vi "Dec 2.vi"() -> ()   [LabVIEW 2020]
uses:
  <vilib>/DAQmx/create/channels.llb/DAQmx Create Channel (AI-Voltage-Basic).vi
  <vilib>/DAQmx/create/scale.llb/DAQmx Create Scale (Linear).vi
  <vilib>/DAQmx/configure/timing.llb/DAQmx Timing (Sample Clock).vi
  <vilib>/DAQmx/read.llb/DAQmx Read (Analog 1D DBL NChan 1Samp).vi
  <vilib>/Utility/file.llb/Write Delimited Spreadsheet (string).vi
  <vilib>/Utility/file.llb/Write Delimited Spreadsheet (DBL).vi
panel:
  in  "stop":bool
  out "Enlapsed Time (sec)":dbl
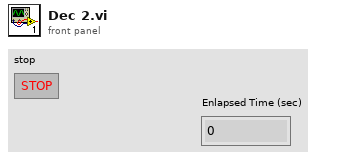
[diagram p1: front panel]
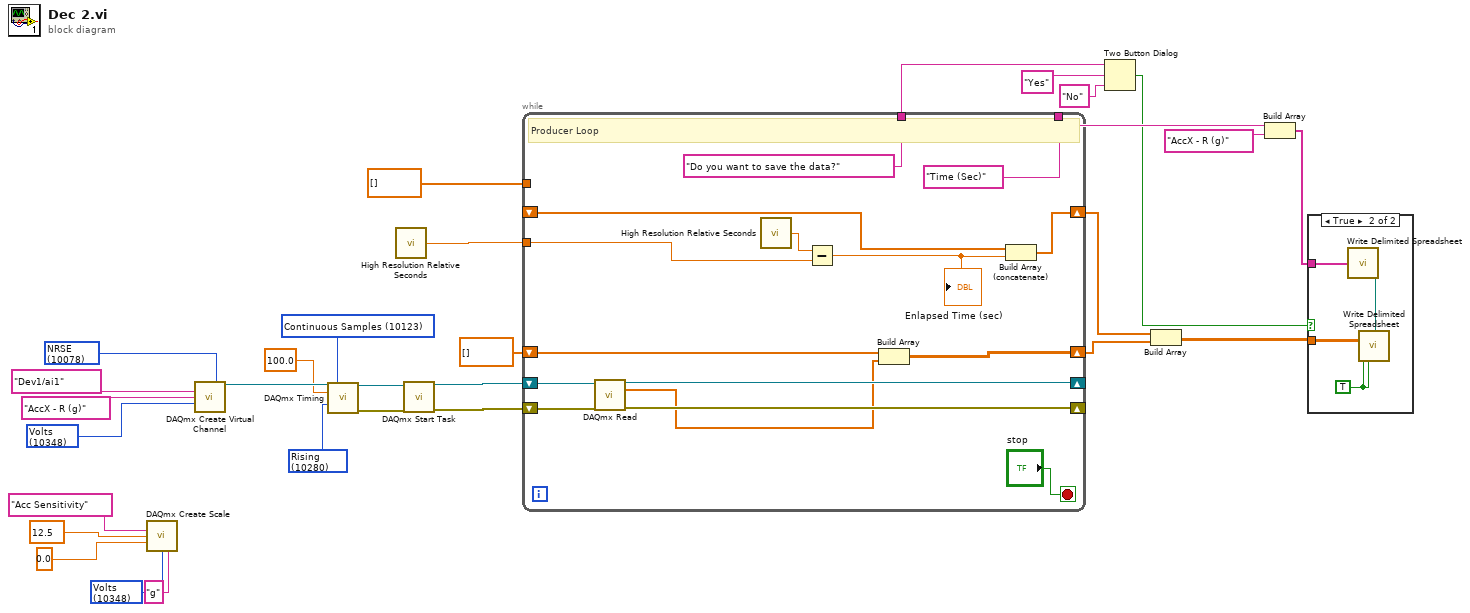
[diagram p0: block diagram]
diagram:
  w18 = 10280 items=["Rising"=10280, "Falling"=10171] ("active edge")
  w19 = 10123 items=["Finite Samples"=10178, "Continuous Samples"=10123, "Hardware Timed Single Point"=12522] ("sample mode")
  w23 = 10348 items=["Volts"=10348, "Amps"=10342, "Deg F"=10144, "Deg C"=10143, "Deg R"=10145, "Kelvins"=10325, "Strain"=10299, "Ohms"=10384, "Hz"=10373, "Seconds"=10364, "Meters"=10219, "Inches"=10379, "Degrees"=10146, "Radians"=10273, "Ticks"=10304, "g"=10186, "m/s^2"=12470, "m/s"=15959, "in/s"=15960, "Pascals"=10081, "Newtons"=15875, "Pounds"=15876, "kgf"=15877, "psi"=15879, "bar"=15880, "Nm"=15881, "oz-in"=15882, "lb-in"=15883, "lb-ft"=15884, "Volts/Volt"=15896, "mVolts/Volt"=15897, "pCoulombs"=16103, "Coulombs"=16102, "From TEDS"=12516] ("pre-scaled units")
  w27 = 10348 items=["Volts"=10348, "From Custom Scale"=10065] ("units")
  w28 = 10078 items=["Default"=-1, "RSE"=10083, "NRSE"=10078, "Differential"=10106, "Pseudodifferential"=12529] ("input terminal configuration")
  n1 = call-poly <vilib>:"DAQmx Create Scale.vi"("name"="Acc Sensitivity", "slope"=12.5, "y-intercept"=0.0, "pre-scaled units"=w23, "scaled units"="g") -> ()  [unwired: 9 in, 2 out]
  n2 = call-poly <vilib>:"DAQmx Create Virtual Channel.vi"("input terminal configuration"=w28, "physical channels"=tag "Dev1/ai1" ("Physical channels"), "name to assign"="AccX - R (g)", "units"=w27) -> ("task out"=w21:refnum<k21>)  [unwired: 10 in, 1 out]
  n3 = call-poly <vilib>:"DAQmx Timing.vi"("task/channels in"=w21, "sample mode"=w19, "rate"=100.0, "active edge"=w18) -> ("task out"=w17:refnum<k21>, "error out"=w16:errorcluster)  [unwired: 10 in]
  n4 = call <vilib>:"High Resolution Relative Seconds.vi"() -> ("relative seconds"=w12:dbl)
  n5 = call <vilib>:"DAQmx Start Task.vi"("task/channels in"=w17, "error in"=w16) -> ("task out"=w15:refnum<k21>, "error out"=w14:errorcluster)  [unwired: 12 in]
  n6 = while {
    shift-right: [w31] -> w10
    shift-left: dbl[] [] -> [w33]
    shift-right: [w41] -> w11
    shift-left: _ -> [w40]
    tunnel: dbl[] [] -> [_]
    tunnel: w12 -> [w39]
    shift-right: [w38] -> _
    shift-left: w14 -> [w44]
    shift-right: [w37] -> _
    shift-left: w15 -> [w45]
    tunnel: ["Time (Sec)"] -> w9
    tunnel: ["Do you want to save the data?" ("message")] -> w2
    stop <- "stop" stop-if-true
    # "Producer Loop"
    n7 = call-poly <vilib>:"DAQmx Read.vi"("task/channels in"=w45, "error in"=w44) -> ("task out"=w37:refnum<k21>, "data"=w32:dbl[], "error out"=w38:errorcluster)  [unwired: 11 in]
    n8 = call <vilib>:"High Resolution Relative Seconds.vi"() -> ("relative seconds"=w43:dbl)
    n9 = Subtract(x=w43, y=w39) -> (x-y=w42:dbl)
    "Enlapsed Time (sec)" <- w42
    n10 = Build Array(w33, w32) -> (w31:dbl[][])
    n11 = Build Array (concatenate)(w40, w42) -> (w41:dbl[])
  }
  n12 = Two Button Dialog(message=w2, 1:"No" ("F button name (\"Cancel\")"), 2:"Yes" ("T button name (\"OK\")")) -> (T button?=w3:bool)
  n13 = Build Array(w11, w10) -> (w7:dbl[][])
  n14 = Build Array(w9, "AccX - R (g)") -> (w8:string[])
  n15 = case shown="True" w3 {
    tunnel: w7 -> [_ w49]
    tunnel: w8 -> [_ w48]
    frame False {
    }
    frame True {
      w47 = TRUE ("transpose? (no:F)")
      n16 = call-poly <vilib>:"Write Delimited Spreadsheet.vi"("1D data"=w48) -> ("new file path (Not A Path if cancelled)"=w46:path)  [unwired: 13 in, 1 out]
      n17 = call-poly <vilib>:"Write Delimited Spreadsheet.vi"("file path (dialog if empty)"=w46, "2D data"=w49, "append to file? (new file:F)"=w47, "transpose? (no:F)"=w47) -> ()  [unwired: 10 in, 2 out]
    }
  }
